vi "Main.vi"(8 "error in":errorcluster, 11 "Controller in":refnum<class "Controller.lvclass">) -> (0 "error out":errorcluster, 3 "Controller out":refnum<class "Controller.lvclass">)   [LabVIEW 2024, in "Controller.lvclass"]
doc: "The <b>Queued Message Handler</b> of the Worker that owns this VI."
uses:
  Controller.lvclass
  Controller.lvclass/Controller.ctl
  Initialization Data.ctl
  Response Cases.ctl
  <vilib>/addons/_Workers/Library/Case Label.ctl
  <vilib>/addons/_Workers/Library/Workers.lvlib
  rqp_Receive CPU Precent.ctl
  CPU Percent/CPU Percent.lvclass
  Place Temperature/Place Temperature.lvclass
  Place Temperature/rqp_Set Place.ctl
  rqp_Receive Temperature.ctl
  Report/Report.lvclass
  Report/rqp_Receive Log Interval.ctl
  rwr_Get Actual Data Reply.ctl
  C:/Program Files (x86)/National Instruments/LabVIEW 2024/vi.lib/addons/_Workers/Library/Classes/Worker/Worker.lvclass
  C:/Program Files (x86)/National Instruments/LabVIEW 2024/vi.lib/addons/_Workers/Library/Classes/Workers Object/Workers Object.lvclass
  C:/_Repo/ugm24-dp2/src/Workers/Controller/Controller.lvclass
  BEEP/BEEP.lvclass
  UGM BEEP/UGM BEEP.lvclass
  UGM BEEP/rqp_UGM BEEP.ctl
panel:
  in  "Log Interval [ms]":i32=2000
  in  "bShowCSV":bool
  in  "Places":string(combo)="Baden, CH"
  out "Temperature":dbl(graph)
  out "Percentage":dbl(graph)
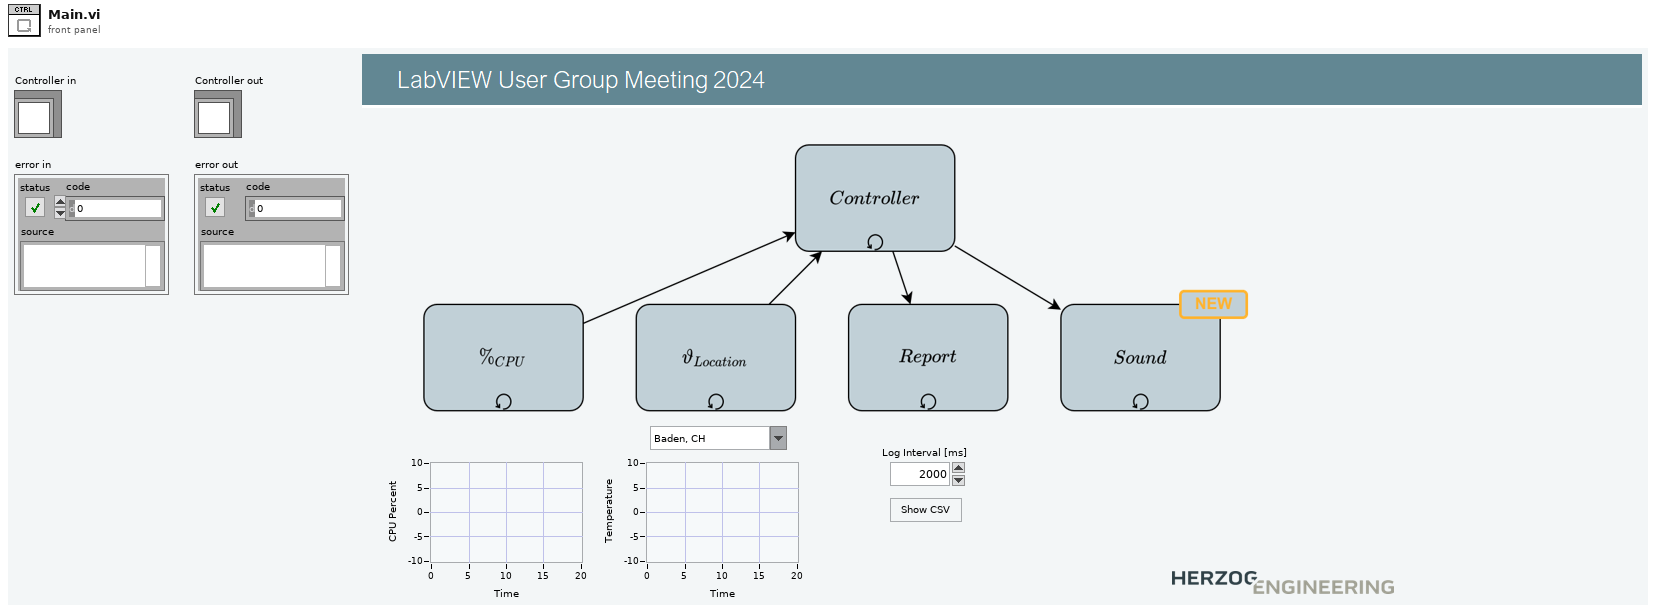
[diagram p1: front panel]
types:
  T1 = typedef "Controller.lvclass/Initialization Data.ctl" = cluster{"Response Cases":T2, "Show Frontpanel":bool}
  T2 = typedef "Controller.lvclass/Response Cases.ctl" = cluster{"Placeholder - Can be deleted":string, "Receive CPU Precent":T3}
  T3 = typedef "Workers.lvlib/Case Label.ctl" = string
  T4 = typedef "Controller.lvclass/rqp_Receive CPU Precent.ctl" = cluster{"CPU Precent":dbl}
  T5 = typedef "Controller.lvclass/rqp_Receive Temperature.ctl" = cluster{"Temperature":dbl}
  T6 = typedef "UGM BEEP.lvclass/rqp_UGM BEEP.ctl" = cluster{"Frequency":u32, "Duration":u32}
  T7 = typedef "Controller.lvclass/rwr_Get Actual Data Reply.ctl" = cluster{"Temperature [°C]":dbl, "CPU [%]":dbl, "Place":string, "Timestamp":timestamp}
  T8 = typedef "Place Temperature.lvclass/rqp_Set Place.ctl" = cluster{"Place":string}
  T9 = typedef "Report.lvclass/rqp_Receive Log Interval.ctl" = cluster{"Interval [ms]":i32}
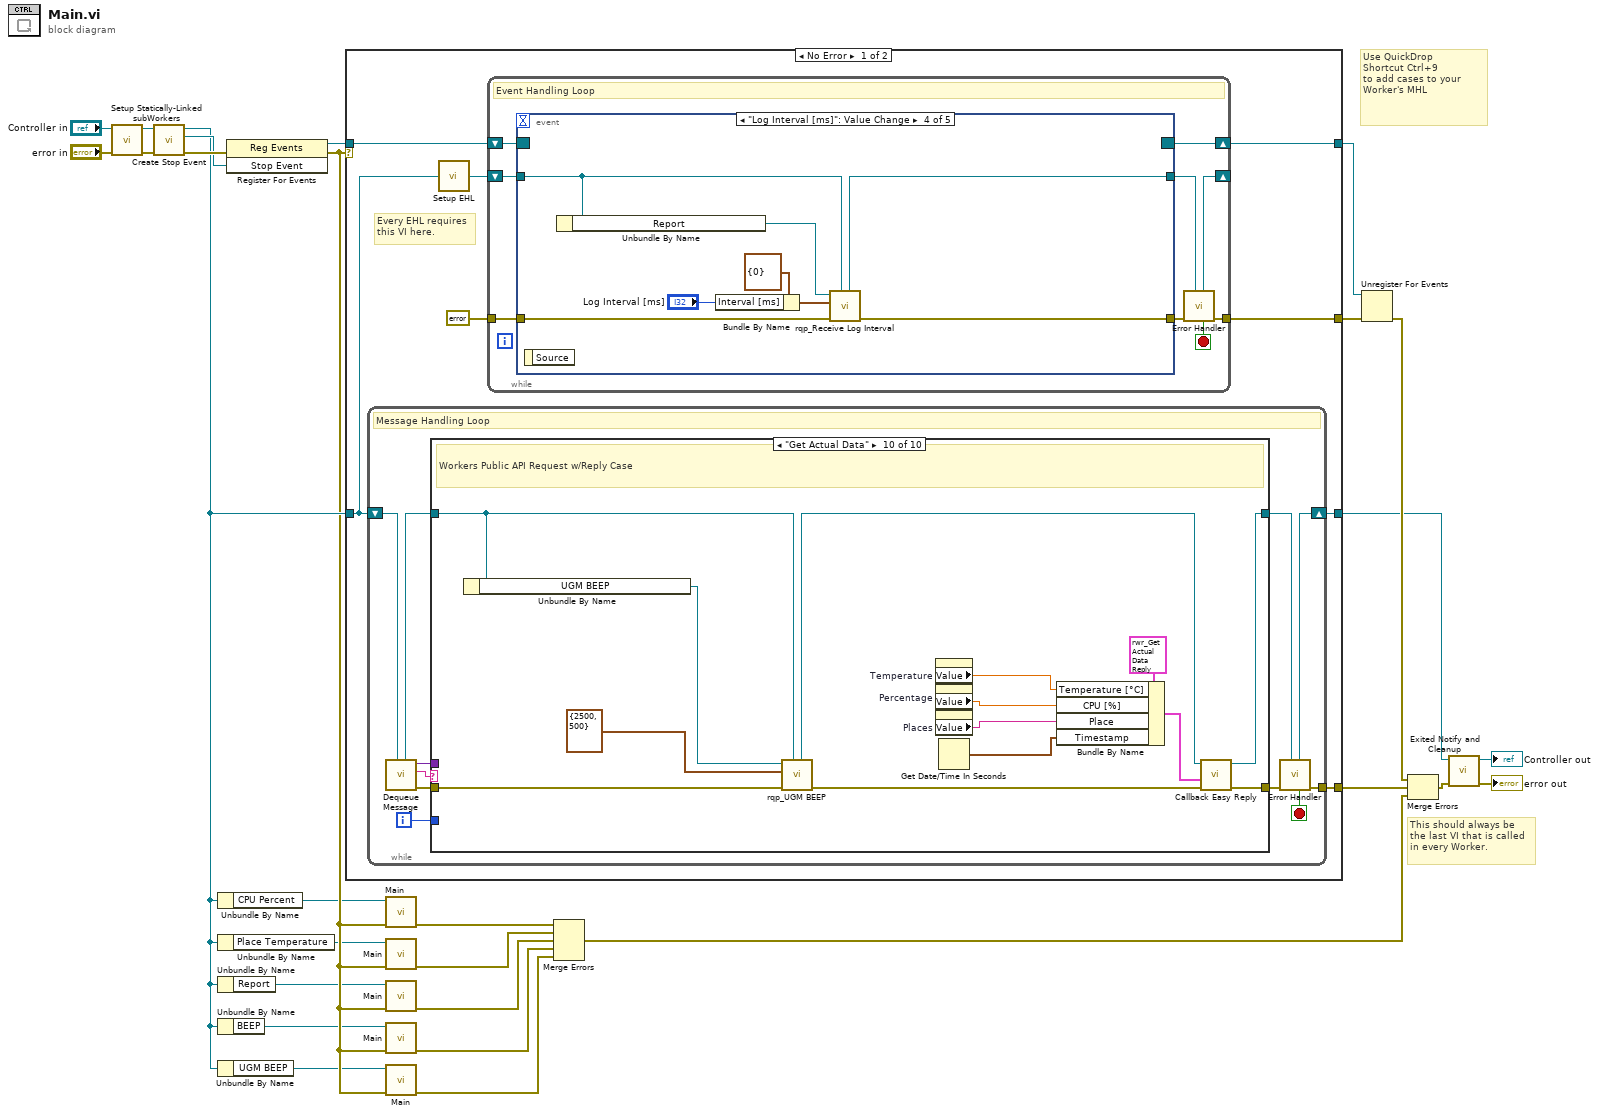
[diagram p0: block diagram]
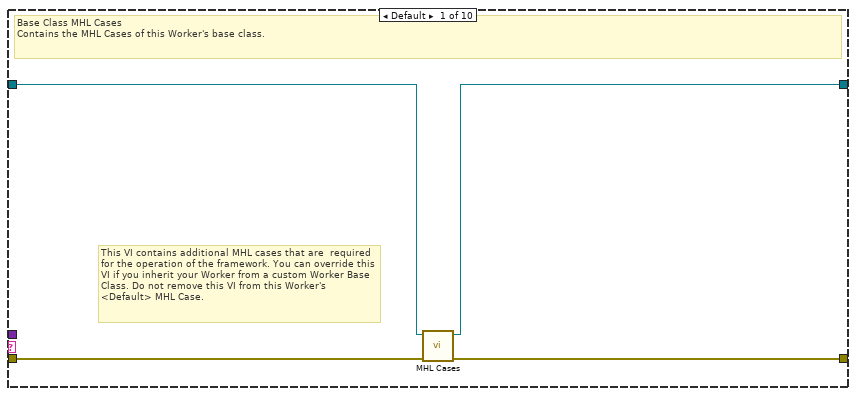
[diagram p2: hidden frame]
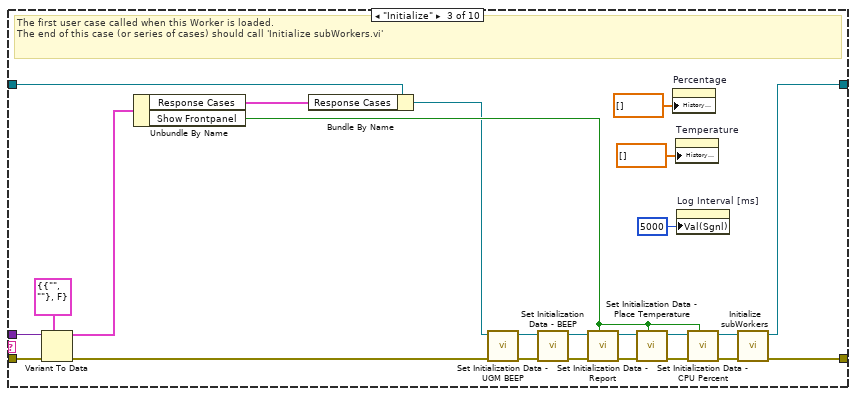
[diagram p4: hidden frame]
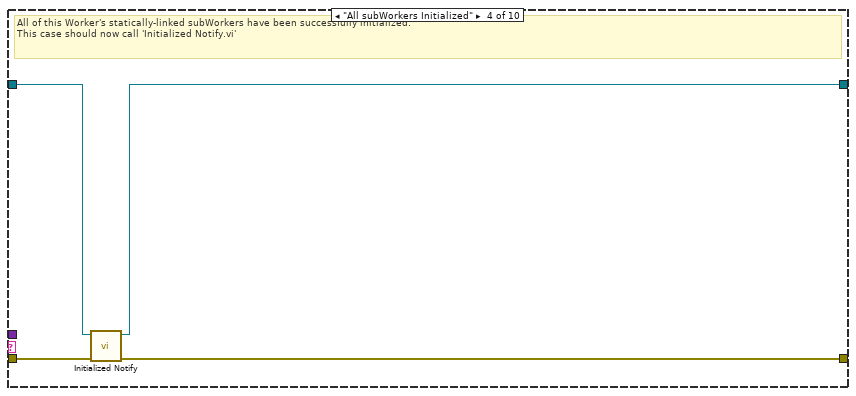
[diagram p5: hidden frame]
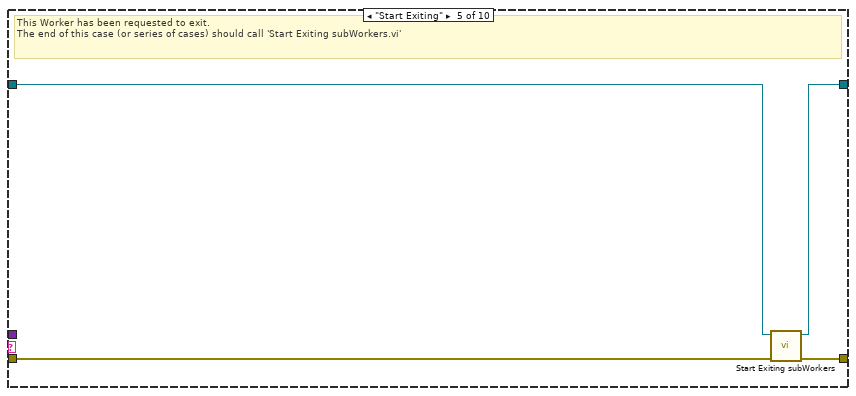
[diagram p6: hidden frame]
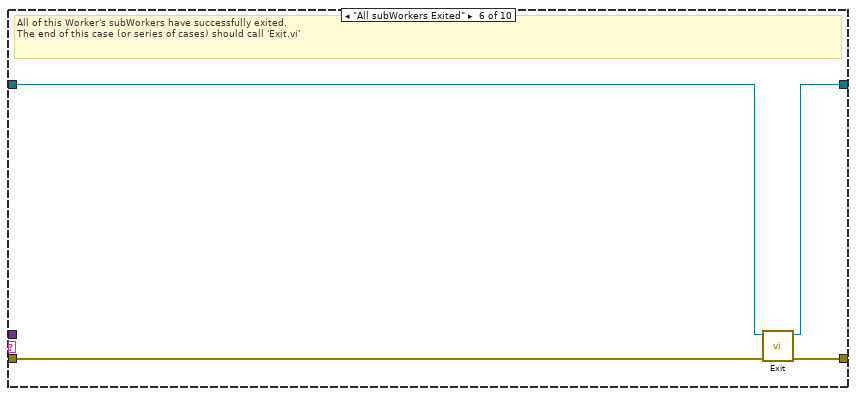
[diagram p7: hidden frame]
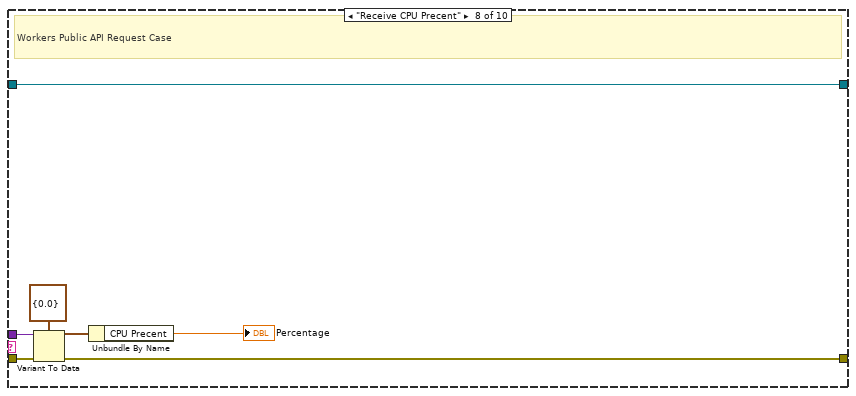
[diagram p9: hidden frame]
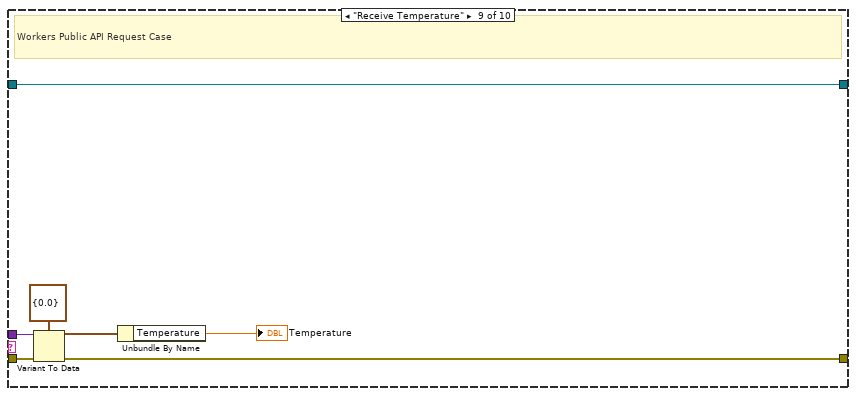
[diagram p10: hidden frame]
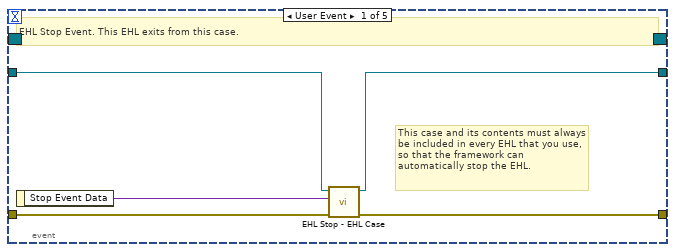
[diagram p11: hidden frame]
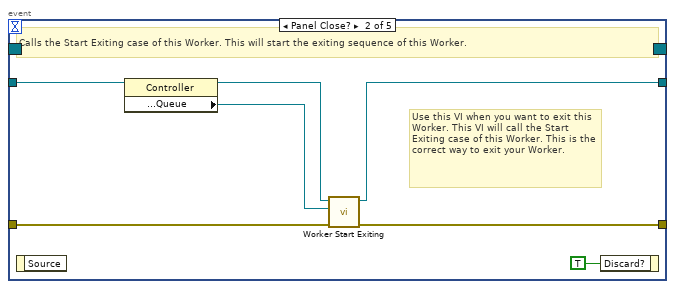
[diagram p12: hidden frame]
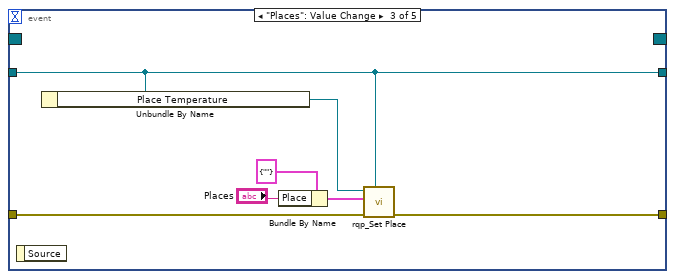
[diagram p13: hidden frame]
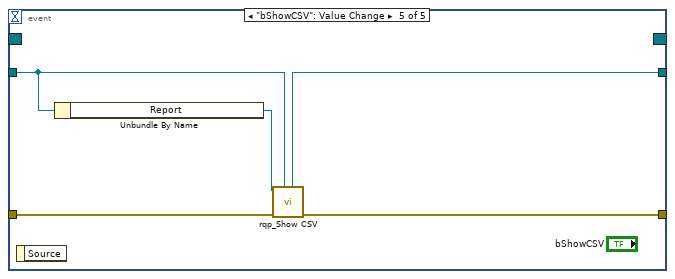
[diagram p14: hidden frame]
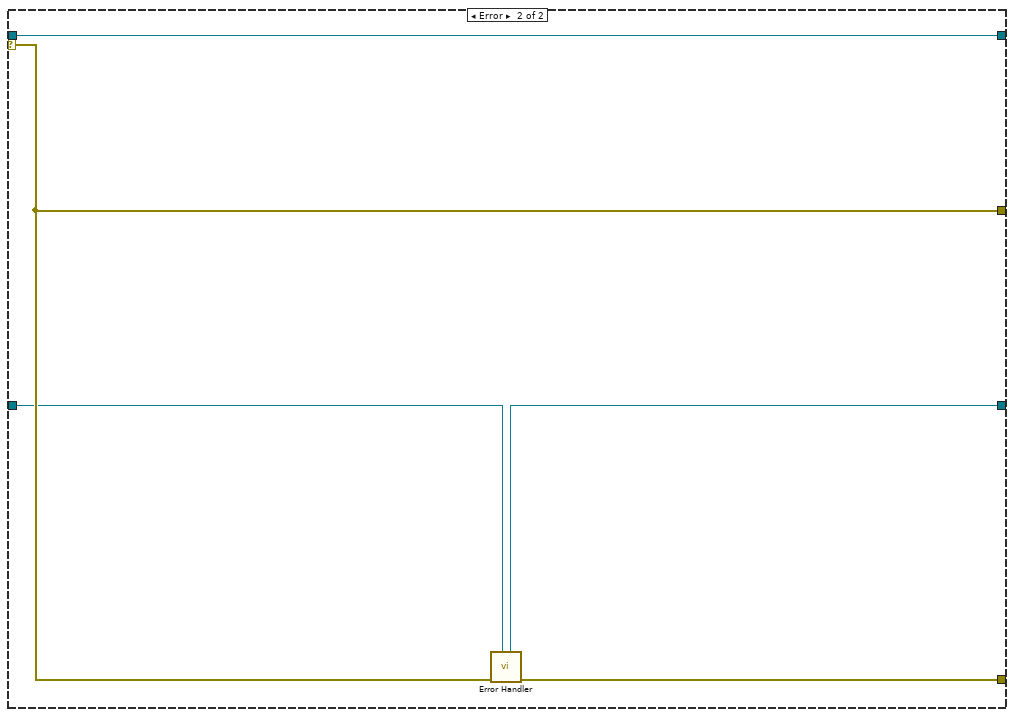
[diagram p15: hidden frame]
diagram:
  # "Use QuickDrop\nShortcut Ctrl+9\nto add cases to your\nWorker's MHL"
  # "This should always be the last VI that is called in every Worker."
  n1 = call "Setup Statically-Linked subWorkers.vi"("error in"="error in", "Controller in"="Controller in") -> ("error out"=w14:errorcluster, "Controller out"=w12:refnum<class "Controller.lvclass">)  [unwired: 8 in]
  n2 = call-dynamic "Create Stop Event.vi"("error in"=w14, "Worker"=w12) -> ("error out"=w23:errorcluster, "Stop Event"=w20:refnum<user-event>, "Worker out"=w17:refnum<class "Controller.lvclass">)  [unwired: 7 in]
  n3 = Unbundle By Name(w17) -> ("CPU Percent"=w9:refnum<class "CPU Percent.lvclass">)
  n4 = Unbundle By Name(w17) -> ("Place Temperature"=w7:refnum<class "Place Temperature.lvclass">)
  n5 = Unbundle By Name(w17) -> ("Report"=w5:refnum<class "Report.lvclass">)
  n6 = Unbundle By Name(w17) -> ("BEEP"=w3:refnum<class "BEEP.lvclass">)
  n7 = Unbundle By Name(w17) -> ("UGM BEEP"=w1:refnum<class "UGM BEEP.lvclass">)
  n8 = register-events(error in=w23, w20) -> (reference out=w22:refnum<event-registration>, error out=w15:errorcluster)  [unwired: 1 in]
  n9 = case shown="No Error" w15 {
    tunnel: w17 -> [w31 w162]
    tunnel: [w29 w163] -> w21
    tunnel: w22 -> [w36 w164]
    tunnel: [w33 w165] -> w27
    tunnel: [w35 w164] -> w26
    tunnel: [w30 w161] -> w24
    selector: w15 -> [_ w165]
    frame No Error {
      # "Every EHL requires\nthis VI here."
      n10 = while {
        shift-right: [w45] -> w30
        shift-left: w31 -> [w47]
        tunnel: [w46] -> w29
        i -> [w38]
        stop <- w39 stop-if-true
        # "Message Handling Loop"
        n11 = call-dynamic "Dequeue Message.vi"("Worker"=w47) -> ("error out"=w44:errorcluster, "Case out"=w40:string, "Data out"=w37:variant, "Worker out"=w42:refnum<class "Controller.lvclass">)  [unwired: 6 in, 1 out]
        n12 = case "Worker MHL Case Structure (DO NOT CHANGE LABEL NAME)" shown="\"Get Actual Data\"" w40 {
          tunnel: w44 -> [w51 w52 w75 w79 w82 w89 w91 w97 w105 w111]
          tunnel: [w50 w52 w77 w78 w85 w88 w91 w96 w104 w119] -> w43
          tunnel: w42 -> [w49 w53 w74 w81 w83 w87 w90 w98 w99 w107]
          tunnel: [w48 w53 w76 w80 w84 w86 w90 w98 w99 w118] -> w41
          tunnel: w38 -> [_ _ _ _ _ _ _ _ _ _]
          tunnel: w37 -> [_ _ w72 _ _ _ _ w94 w102 _]
          frame Default {
            # "This VI contains additional MHL cases that are  required for the operation of the framework. You can override this VI if you inherit your Worker from a custom Worker Base Class. Do not remove this VI from this Worker's <Default> MHL Case."
            # "Base Class MHL Cases\nContains the MHL Cases of this Worker's base class."
            n13 = call-dynamic "MHL Cases.vi"("error in"=w51, "Worker in"=w49) -> ("error out"=w50:errorcluster, "Worker out"=w48:refnum<class "Controller.lvclass">)  [unwired: 8 in]
          }
          frame "------------ FRAMEWORK CASES -----------" {
            # "Start of Workers Framework Cases"
          }
          frame "Initialize" {
            # "The first user case called when this Worker is loaded.\nThe end of this case (or series of cases) should call 'Initialize subWorkers.vi'"
            n14 = Variant To Data(error in=w75, type=T1 {"Response Cases"={"Placeholder - Can be deleted"="", "Receive CPU Precent"=""}, "Show Frontpanel"=FALSE} ("Initialization Data"), Variant=w72) -> (data=w71:T1, error out=w73:errorcluster)
            n15 = Unbundle By Name(w71) -> ("Response Cases"=w70:T2, "Show Frontpanel"=w58:bool)
            n16 = Bundle By Name(cluster=w74, "Response Cases"=w70) -> (w55:refnum<class "Controller.lvclass">)
            n17 = call "Set Initialization Data - UGM BEEP.vi"("error in"=w73, "Controller in"=w55) -> ("error out"=w56:errorcluster, "Controller out"=w54:refnum<class "Controller.lvclass">)  [unwired: 8 in]
            n18 = call "Set Initialization Data - BEEP.vi"("error in"=w56, "Controller in"=w54) -> ("error out"=w60:errorcluster, "Controller out"=w59:refnum<class "Controller.lvclass">)  [unwired: 8 in]
            n19 = call "Set Initialization Data - Report.vi"("Show Frontpanel"=w58, "error in"=w60, "Controller in"=w59) -> ("error out"=w62:errorcluster, "Controller out"=w61:refnum<class "Controller.lvclass">)  [unwired: 7 in]
            n20 = call "Set Initialization Data - Place Temperature.vi"("Show Frontpanel"=w58, "error in"=w62, "Controller in"=w61) -> ("error out"=w66:errorcluster, "Controller out"=w65:refnum<class "Controller.lvclass">)  [unwired: 7 in]
            n21 = property on="Percentage" class="WFChart (strict)"("History Data"=dbl[] []) -> ()  [unwired: 2 in, 2 out]
            n22 = property on="Temperature" class="WFChart (strict)"("History Data"=dbl[] []) -> ()  [unwired: 2 in, 2 out]
            n23 = property on="Log Interval [ms]" class="DigNum (strict)"("Val(Sgnl)"=5000 ("Value (Signaling)")) -> ()  [unwired: 2 in, 2 out]
            n24 = call "Set Initialization Data - CPU Percent.vi"("Show Frontpanel"=w58, "error in"=w66, "Controller in"=w65) -> ("error out"=w68:errorcluster, "Controller out"=w67:refnum<class "Controller.lvclass">)  [unwired: 7 in]
            n25 = call-dynamic "Initialize subWorkers.vi"("error in"=w68, "Worker"=w67) -> ("error out"=w77:errorcluster, "dup Worker out"=w76:refnum<class "Controller.lvclass">)  [unwired: 8 in]
          }
          frame "All subWorkers Initialized" {
            # "All of this Worker's statically-linked subWorkers have been successfully initialized.\nThis case should now call 'Initialized Notify.vi'"
            n26 = call-dynamic "Initialized Notify.vi"("error in"=w79, "Worker"=w81) -> ("error out"=w78:errorcluster, "dup Worker out"=w80:refnum<class "Controller.lvclass">)  [unwired: 8 in]
          }
          frame "Start Exiting" {
            # "This Worker has been requested to exit. \nThe end of this case (or series of cases) should call 'Start Exiting subWorkers.vi'"
            n27 = call-dynamic "Start Exiting subWorkers.vi"("error_in"=w82, "Worker"=w83) -> ("error out"=w85:errorcluster, "dup Worker out"=w84:refnum<class "Controller.lvclass">)  [unwired: 8 in]
          }
          frame "All subWorkers Exited" {
            # "All of this Worker's subWorkers have successfully exited. \nThe end of this case (or series of cases) should call 'Exit.vi'"
            n28 = call-dynamic "Exit.vi"("error_in"=w89, "Worker"=w87) -> ("error out"=w88:errorcluster, "dup Worker out"=w86:refnum<class "Controller.lvclass">)  [unwired: 8 in]
          }
          frame "------------- PUBLIC API CASES -------------" {
            # "Start of Workers Public API Cases"
          }
          frame "Receive CPU Precent" {
            # "Workers Public API Request Case"
            n29 = Variant To Data(error in=w97, type=T4 {"CPU Precent"=0.0} ("Data"), Variant=w94) -> (data=w93:T4, error out=w96:errorcluster)
            n30 = Unbundle By Name(w93) -> ("CPU Precent"=→"Percentage":dbl)
          }
          frame "Receive Temperature" {
            # "Workers Public API Request Case"
            n31 = Variant To Data(error in=w105, type=T5 {"Temperature"=0.0} ("Data"), Variant=w102) -> (data=w101:T5, error out=w104:errorcluster)
            n32 = Unbundle By Name(w101) -> ("Temperature"=→"Temperature":dbl)
          }
          frame "Get Actual Data" {
            # "Workers Public API Request w/Reply Case"
            n33 = Unbundle By Name(w107) -> ("UGM BEEP"=w109:refnum<class "UGM BEEP.lvclass">)
            n34 = call "rqp_UGM BEEP.vi"("Caller in"=w107, "error in"=w111, "Data in"=T6 {"Frequency"=2500, "Duration"=500}, "UGM BEEP in"=w109) -> ("error out"=w110:errorcluster, "dup Caller out"=w108:refnum<class "Controller.lvclass">)  [unwired: 5 in, 1 out]
            n35 = property on="Temperature" class="WFChart (strict)"() -> ("Value"=w115:dbl)  [unwired: 2 in, 2 out]
            n36 = property on="Percentage" class="WFChart (strict)"() -> ("Value"=w114:dbl)  [unwired: 2 in, 2 out]
            n37 = property on="Places" class="CmbBox"() -> ("Value"=w113:string)  [unwired: 2 in, 2 out]
            n38 = Get Date/Time In Seconds() -> (seconds since 1Jan1904=w112:timestamp)
            n39 = Bundle By Name(cluster=T7 {"Temperature [°C]"=0.0, "CPU [%]"=0.0, "Place"="", "Timestamp"=timestamp(0 s since 1904-01-01)} ("Reply Data"), "Temperature [°C]"=w115, "CPU [%]"=w114, "Place"=w113, "Timestamp"=w112) -> (w116:T7)
            n40 = call-dynamic "Callback Easy Reply.vi"("error in"=w110, "Data"=w116, "Worker"=w108) -> ("error out"=w119:errorcluster, "dup Worker out"=w118:refnum<class "Controller.lvclass">)  [unwired: 7 in]
          }
        }
        n41 = call-dynamic "Error Handler.vi"("Worker"=w41, "error_in"=w43) -> ("error out"=w46:errorcluster, "Stop Loop"=w39:bool, "Worker out"=w45:refnum<class "Controller.lvclass">)  [unwired: 7 in]
      }
      n42 = call-dynamic "Setup EHL.vi"("Worker"=w31) -> ("Worker out"=w32:refnum<class "Controller.lvclass">)  [unwired: 14 in]
      n43 = while "Event Handling Loop" {
        shift-right: [w128] -> w35
        shift-left: w36 -> [w127]
        tunnel: [w123] -> w33
        tunnel: errorcluster {"status"=FALSE, "code"=0, "source"=""} ("error constant") -> [w125]
        shift-right: [w121] -> _
        shift-left: w32 -> [w126]
        stop <- w120 stop-if-true
        # "Event Handling Loop"
        n44 = event shown="[3] \"Log Interval [ms]\": Value Change" {
          selector: w127 -> [_ _ _ _ _]
          dyn-events: [_ _ _ _ _] -> w128
          timeout: _ -> [_ _ _ _ _]
          tunnel: [w132 w139 w143 w154 w159] -> w124
          tunnel: w125 -> [w133 w138 w144 w155 w160]
          tunnel: w126 -> [w131 w137 w142 w152 w157]
          tunnel: [w130 w136 w142 w153 w158] -> w122
          event User Event {
            # "This case and its contents must always be included in every EHL that you use, so that the framework can automatically stop the EHL."
            # "EHL Stop Event. This EHL exits from this case."
            n45 = event-data() -> ("Stop Event Data"=w129:variant)  [unwired: 1 in]
            n46 = call-dynamic "EHL Stop - EHL Case.vi"("error in"=w133, "Stop Event Data"=w129, "Worker"=w131) -> ("error out"=w132:errorcluster, "Worker out"=w130:refnum<class "Controller.lvclass">)  [unwired: 7 in]
          }
          event Panel Close? {
            # "Use this VI when you want to exit this Worker. This VI will call the Start Exiting case of this Worker. This is the correct way to exit your Worker."
            # "Calls the Start Exiting case of this Worker. This will start the exiting sequence of this Worker."
            n47 = event-data() -> ()  [unwired: 1 in, 1 out]
            n48 = property class="Controller"(reference=w137) -> (reference out=w135:refnum<class "Controller.lvclass">, "Accessors:Read:Public API:Queue"=w134:refnum<class "Message Queue.lvclass">)  [unwired: 1 in, 1 out]
            n49 = call-dynamic "Worker Start Exiting.vi"("error_in"=w138, "Message Queue"=w134, "Worker"=w135) -> ("error out"=w139:errorcluster, "dup Worker out"=w136:refnum<class "Controller.lvclass">)  [unwired: 7 in]
            n50 = event-data ("Event Filter Node")("Discard?"=TRUE) -> ()  [unwired: 1 in, 1 out]
          }
          event "Places": Value Change {
            n51 = event-data() -> ()  [unwired: 1 in, 1 out]
            n52 = Unbundle By Name(w142) -> ("Place Temperature"=w141:refnum<class "Place Temperature.lvclass">)
            n53 = Bundle By Name(cluster=T8 {"Place"=""} ("Data in"), "Place"="Places") -> (w146:T8)
            n54 = call "rqp_Set Place.vi"("Caller in"=w142, "error in"=w144, "Data in"=w146, "Place Temperature in"=w141) -> ("error out"=w143:errorcluster)  [unwired: 5 in, 2 out]
          }
          event "Log Interval [ms]": Value Change {
            n55 = event-data() -> ()  [unwired: 1 in, 1 out]
            n56 = Unbundle By Name(w152) -> ("Report"=w151:refnum<class "Report.lvclass">)
            n57 = Bundle By Name(cluster=T9 {"Interval [ms]"=0} ("Data in"), "Interval [ms]"="Log Interval [ms]") -> (w150:T9)
            n58 = call "rqp_Receive Log Interval.vi"("Caller in"=w152, "error in"=w155, "Data in"=w150, "Report in"=w151) -> ("error out"=w154:errorcluster, "dup Caller out"=w153:refnum<class "Controller.lvclass">)  [unwired: 5 in, 1 out]
          }
          event "bShowCSV": Value Change {
            n59 = event-data() -> ()  [unwired: 1 in, 1 out]
            n60 = Unbundle By Name(w157) -> ("Report"=w156:refnum<class "Report.lvclass">)
            n61 = call "rqp_Show CSV.vi"("Caller in"=w157, "error in"=w160, "Report in"=w156) -> ("error out"=w159:errorcluster, "dup Caller out"=w158:refnum<class "Controller.lvclass">)  [unwired: 6 in, 1 out]
          }
        }
        n62 = call-dynamic "Error Handler.vi"("Worker"=w122, "error_in"=w124) -> ("error out"=w123:errorcluster, "Stop Loop"=w120:bool, "Worker out"=w121:refnum<class "Controller.lvclass">)  [unwired: 7 in]
      }
    }
    frame Error {
      n63 = call-dynamic "Error Handler.vi"("Worker"=w162, "error_in"=w165) -> ("error out"=w163:errorcluster, "Worker out"=w161:refnum<class "Controller.lvclass">)  [unwired: 7 in, 1 out]
    }
  }
  n64 = call-dynamic "Main.vi"("error in"=w15, "CPU Percent in"=w9) -> ("error out"=w11:errorcluster)  [unwired: 8 in, 1 out]
  n65 = call-dynamic "Main.vi"("error in"=w15, "CPU Percent in"=w7) -> ("error out"=w8:errorcluster)  [unwired: 8 in, 1 out]
  n66 = call-dynamic "Main.vi"("error in"=w15, "Report in"=w5) -> ("error out"=w6:errorcluster)  [unwired: 8 in, 1 out]
  n67 = call-dynamic "Main.vi"("error in"=w15, "BEEP in"=w3) -> ("error out"=w4:errorcluster)  [unwired: 8 in, 1 out]
  n68 = call-dynamic "Main.vi"("error in"=w15, "UGM BEEP in"=w1) -> ("error out"=w2:errorcluster)  [unwired: 8 in, 1 out]
  n69 = Merge Errors(w11, w8, w6, w4, w2) -> (w10:errorcluster)
  n70 = Unregister For Events(event registration refnum=w26, error in=w27) -> (error out=w28:errorcluster)
  n71 = Merge Errors(w28, w21, w10) -> (w25:errorcluster)
  n72 = call-dynamic "Exited Notify and Cleanup.vi"("error_in"=w25, "Worker"=w24) -> ("error out"=→"error out":errorcluster, "dup Worker out"=→"Controller out":refnum<class "Controller.lvclass">)  [unwired: 8 in]
